vi "Main_System.vi"(11 "LabVIEW Web Service Request":refnum<class "Web Request.lvclass">=refnum) -> ()   [LabVIEW 2017]
uses:
  <vilib>/wsapi/Web Request.lvclass
  TypeDef/RF_StateMachine.ctl
panel:
  in  "Tab Control":enum32{"Basic UI", "Debug"}(tab)
  out "Test Progress":dbl(slide) max=6.0 step=1.0 scale=0.0..100.0
  out "Status (error)":bool
  out "Playback Progress":i32(slide)=383 scale=-1.0..536.0
  out "error out":errorcluster
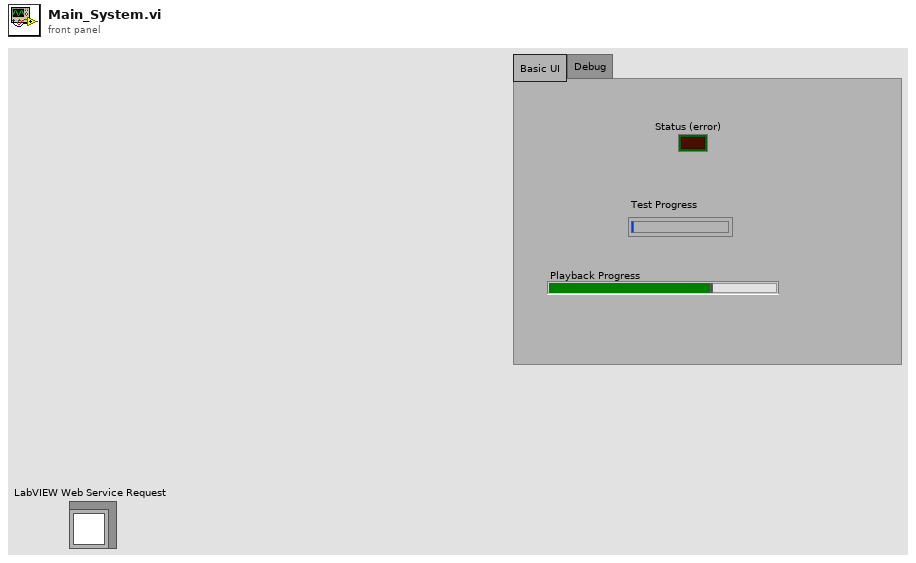
[diagram p1: front panel]
types:
  T1 = typedef "RF_StateMachine.ctl" = enum16{"Parse Metadata", "Convert File", "Play File", "Finished Playing", "Send Message", "Report Error", "Exit"}
  T2 = typedef "ESC Internal Data Structure (types).ctl" = cluster{"Test_File":path, "Status":string, "RF_Center_Freq":dbl, "RF_Gain":dbl, "BB_Gain":dbl, "Error 2":string, "file_max":u64, "file_index":u64}
  T3 = typedef "RF Internal Data Structure (string).ctl" = cluster{"Test_File":string, "Status":string, "RF_Center_Freq":string, "RF_Gain":string, "BB_Gain":string, "Error":string, "file_max":string, "file_index":string}
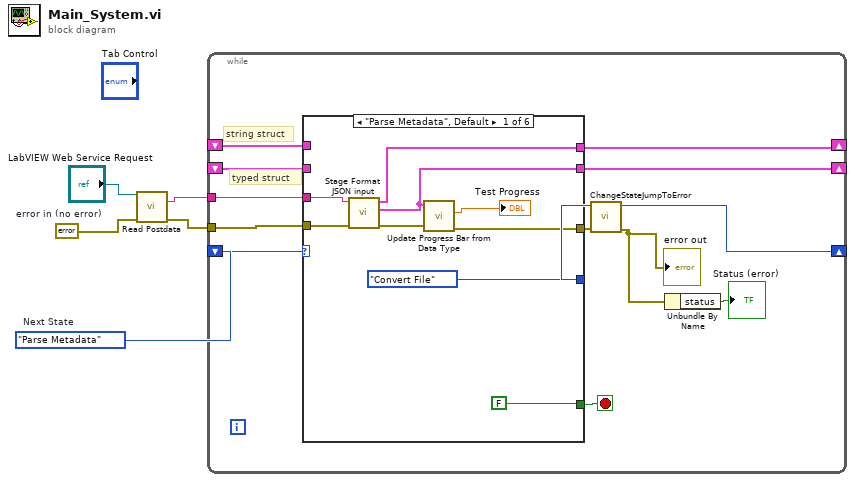
[diagram p0: block diagram]
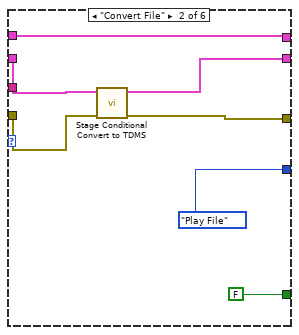
[diagram p2: hidden frame]
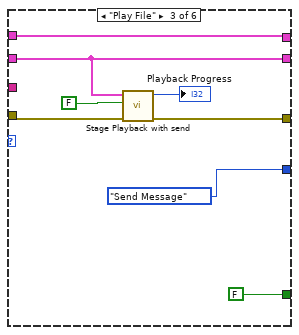
[diagram p3: hidden frame]
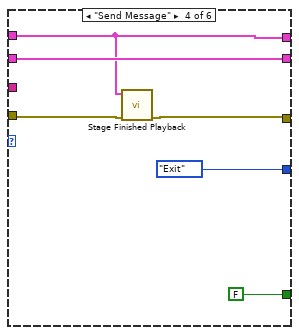
[diagram p4: hidden frame]
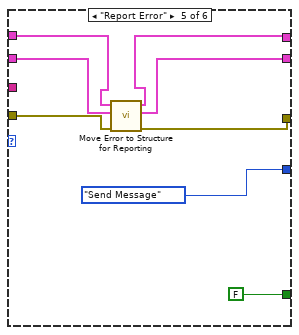
[diagram p5: hidden frame]
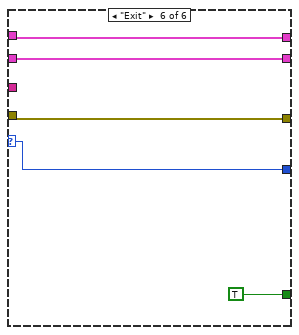
[diagram p6: hidden frame]
diagram:
  w2 = RF_StateMachine."Parse Metadata"  # Next State
  w4 = errorcluster {"status"=FALSE, "code"=0, "source"=""}  # error in (no error)
  n1 = call <vilib>:"Read Postdata.vi"("LabVIEW Web Service Request"="LabVIEW Web Service Request", "error in (no error)"=w4) -> ("postdata"=w1:string, "error out"=w3:errorcluster)  [unwired: 11 in, 1 out]
  n2 = while {
    tunnel: w3 -> [w17]
    shift-right: [w11] -> _
    shift-left: w2 -> [w10]
    shift-right: [w14] -> _
    shift-left: _ -> [w8]
    shift-right: [w15] -> _
    shift-left: _ -> [w7]
    tunnel: w1 -> [w9]
    stop <- w16 stop-if-true
    # "typed struct"
    # "string struct"
    n3 = case shown="\"Parse Metadata\", Default" w10 {
      selector: w10 -> [_ _ _ _ _ w57]
      tunnel: [w26 w33 w39 w44 w49 w58] -> w18
      tunnel: [w20 w34 w41 w46 w51 w59] -> w15
      tunnel: [w25 w28 w42 w43 w52 w60] -> w14
      tunnel: w17 -> [w24 w32 w40 w45 w50 w58]
      tunnel: [FALSE FALSE FALSE FALSE FALSE TRUE] -> w16
      tunnel: w9 -> [w22 _ _ _ _ _]
      tunnel: w8 -> [_ w28 w42 w43 w53 w60]
      tunnel: w7 -> [_ w31 w41 w46 w54 w59]
      tunnel: [RF_StateMachine."Convert File" ("Next State (pre error check)") RF_StateMachine."Play File" ("Next State (pre error check)") RF_StateMachine."Send Message" ("Next State (pre error check)") RF_StateMachine."Exit" ("Next State (pre error check)") RF_StateMachine."Send Message" ("Next State (pre error check)") w57] -> w6
      frame "Parse Metadata", Default {
        n4 = call "Stage Format JSON input.vi"("error in (no error)"=w24, "JSON string (in)"=w22) -> ("error out"=w27:errorcluster, "ESC Internal Data Structure (with types)"=w20:T2, "Internal Vars"=w25:T3)  [unwired: 7 in]
        n5 = call "Update Progress Bar from Data Type.vi"("error in"=w27, "ESC Internal Data Structure (with types)"=w20) -> ("error out"=w26:errorcluster, "Test Progress"=→"Test Progress":dbl)  [unwired: 7 in, 1 out]
      }
      frame "Convert File" {
        n6 = call "Stage Conditional Convert to TDMS.vi"("error in (no error)"=w32, "input cluster"=w31) -> ("error out"=w33:errorcluster, "output cluster"=w34:T2)  [unwired: 7 in, 1 out]
      }
      frame "Play File" {
        n7 = call "Stage Playback with send.vi"("error in (no error)"=w40, "IQ Swap Enabled"=FALSE ("use V2"), "input cluster"=w41) -> ("error out"=w39:errorcluster, "Playback Progress"=→"Playback Progress":i32)  [unwired: 6 in, 1 out]
      }
      frame "Send Message" {
        n8 = call "Stage Finished Playback.vi"("error in (no error)"=w45, "Internal Vars"=w43) -> ("error out"=w44:errorcluster)  [unwired: 9 in]
      }
      frame "Report Error" {
        n9 = call "Move Error to Structure for Reporting.vi"("error in (expected)"=w50, "ESC Internal Data Structure (with types)"=w54, "ESC Internal Data Structure (with strings)"=w53) -> ("error out"=w49:errorcluster, "ESC Internal Data Structure (with types) out"=w51:T2, "ESC Internal Data Structure (with strings) out"=w52:T3)  [unwired: 6 in]
      }
      frame "Exit" {
      }
    }
    n10 = call "ChangeStateJumpToError.vi"("err in"=w18, "Next State (pre error check)"=w6) -> ("err out"=w12:errorcluster, "Next State (post error check)"=w11:T1)  [unwired: 8 in]
    "error out" <- w12
    n11 = Unbundle By Name(w12) -> ("status"=→"Status (error)":bool)
  }
